vi "Initialize WORD.vi"(8 "error in (no error)":errorcluster, 11 "NI_report in":refnum<class "NI_report.lvclass">) -> (0 "error out":errorcluster, 3 "NI_report out":refnum<class "NI_report.lvclass">)   [LabVIEW 2015, in "Report.lvlib"]
uses:
  Report.lvlib
  <vilib>/Utility/NIReport.llb/NI_report.lvclass
  <vilib>/Utility/NIReport.llb/Append Report Text (str wrap).vi
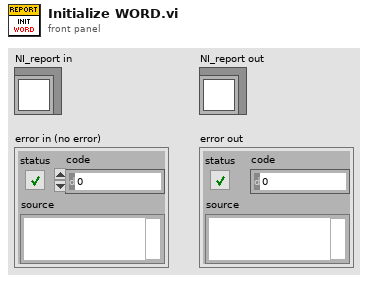
[diagram p1: front panel]
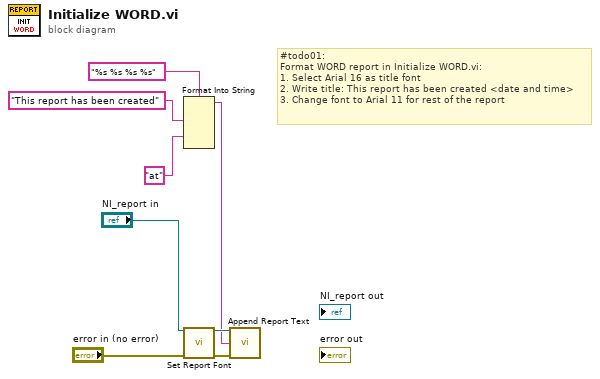
[diagram p0: block diagram]
diagram:
  # "#todo01:\nFormat WORD report in Initialize WORD.vi:\n1. Select Arial 16 as title font\n2. Write title: This report has been created <date and time>\n3. Change font to Arial 11 for rest of the report"
  n1 = Format Into String(format string="%s %s %s %s", "This report has been created" ("input 1"), "at" ("input 3")) -> (resulting string=w4:string)  [unwired: 4 in, 1 out]
  n2 = call-dynamic "Set Report Font.vi"("report in"="NI_report in", "error in (no error)"="error in (no error)") -> ("report out"=w7:refnum<class "NI_report.lvclass">, "error out"=w8:errorcluster)  [unwired: 11 in, 1 out]
  n3 = call-poly <vilib>:"Append Report Text.vi"("report in"=w7, "text"=w4, "error in (no error)"=w8) -> ()  [unwired: 9 in, 4 out]
